vi "gun_auton_custom_shot.vi"(10 "data_store_mode":enum16{"Set", "Get"}(ring), 11 "shot params":T1) -> (3 "shot params out":T1)   [LabVIEW 2011]
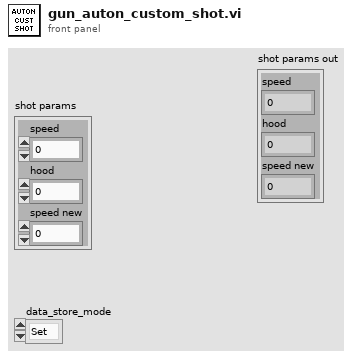
[diagram p1: front panel]
types:
  T1 = cluster{"speed":dbl, "hood":dbl, "speed new":dbl}
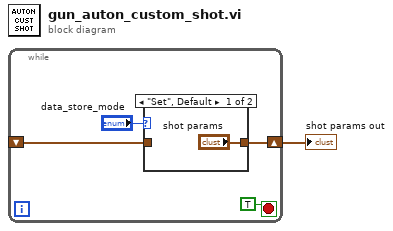
[diagram p0: block diagram]
diagram:
  n1 = while {
    shift-right: [w3] -> w1
    shift-left: _ -> [w2]
    stop <- TRUE stop-if-true
    n2 = case shown="\"Set\", Default" "data_store_mode" {
      tunnel: ["shot params" w7] -> w3
      tunnel: w2 -> [_ w7]
      frame "Set", Default {
      }
      frame "Get" {
      }
    }
  }
  "shot params out" <- w1
